vi "Initialize_Images_Array_Random_Names-1.vi"(2 "error IN":errorcluster, 3 "[IN] # Pics":i32, 4 "[IN] Image Type":T1 items=["Grayscale (U8)", "Grayscale (I16)", "Grayscale (SGL)", "Complex (CSG)", "RGB (U32)", "HSL (U32)", "RGB (U64)", "Grayscale (U16)"]) -> (0 "error OUT":errorcluster, 1 "[OUT] Images Array":T2[](array[typedef]))   [LabVIEW 2017]
doc: "Produces the pre-allocated array with initialized references to images"
uses:
  <vilib>/vision/Image Controls.llb/IMAQ Image.ctl
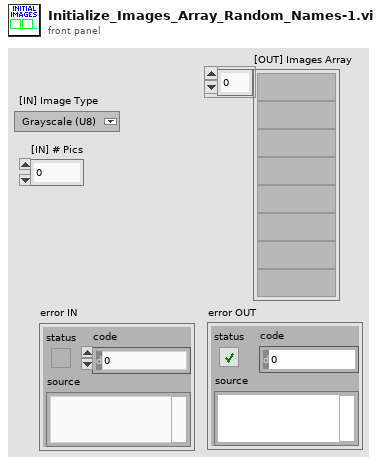
[diagram p1: front panel]
types:
  T1 = typedef "Image Type" = u32
  T2 = typedef "IMAQ Image.ctl" = refnum<image>
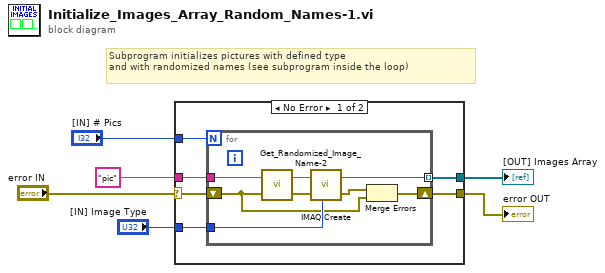
[diagram p0: block diagram]
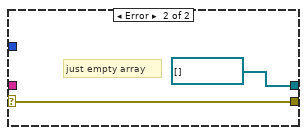
[diagram p2: hidden frame]
diagram:
  # "Subprogram initializes pictures with defined type \nand with randomized names (see subprogram inside the loop)"
  n1 = case shown="No Error" "error IN" {
    selector: "error IN" -> [w8 w22]
    tunnel: "[IN] Image Type" -> [w12 _]
    tunnel: [w11 T2[] []] -> w5
    tunnel: "pic" ("Main Name") -> [w10 _]
    tunnel: "[IN] # Pics" -> [w9 _]
    tunnel: [w7 w22] -> w1
    frame No Error {
      n2 = for {
        N: w9 -> [_]
        tunnel: [w20] -> w11 mode=indexing
        tunnel: w12 -> [w19]
        tunnel: w10 -> [w18]
        shift-right: [w15] -> w7
        shift-left: w8 -> [w13]
        n3 = call "Get_Randomized_Image_Name-2.vi"("error IN"=w13, "[IN] Main Name"=w18) -> ("error OUT"=w16:errorcluster, "[OUT] Randomized name"=w17:string)
        n4 = call "IMAQ Create"("Image Name"=w17, "Image Type"=w19, "error in (no error)"=w16) -> ("New Image"=w20:T2, "error out"=w14:errorcluster)  [unwired: 2 in]
        n5 = Merge Errors(w14, w13) -> (w15:errorcluster)
      }
    }
    frame Error {
      # "just empty array"
    }
  }
  "[OUT] Images Array" <- w5
  "error OUT" <- w1
